vi "Middfield_171213.vi"(8 "StartingAngle":i16, 9 "DiameterOfTheMidfield":u16, 10 "Midfield":enum16{"4", "3", "2", "1", "0"}(ring), 11 "InputBackground":picture) -> (2 "Colors":u32[](array[numeric]), 3 "OutputBackground":picture)   [LabVIEW 2016]
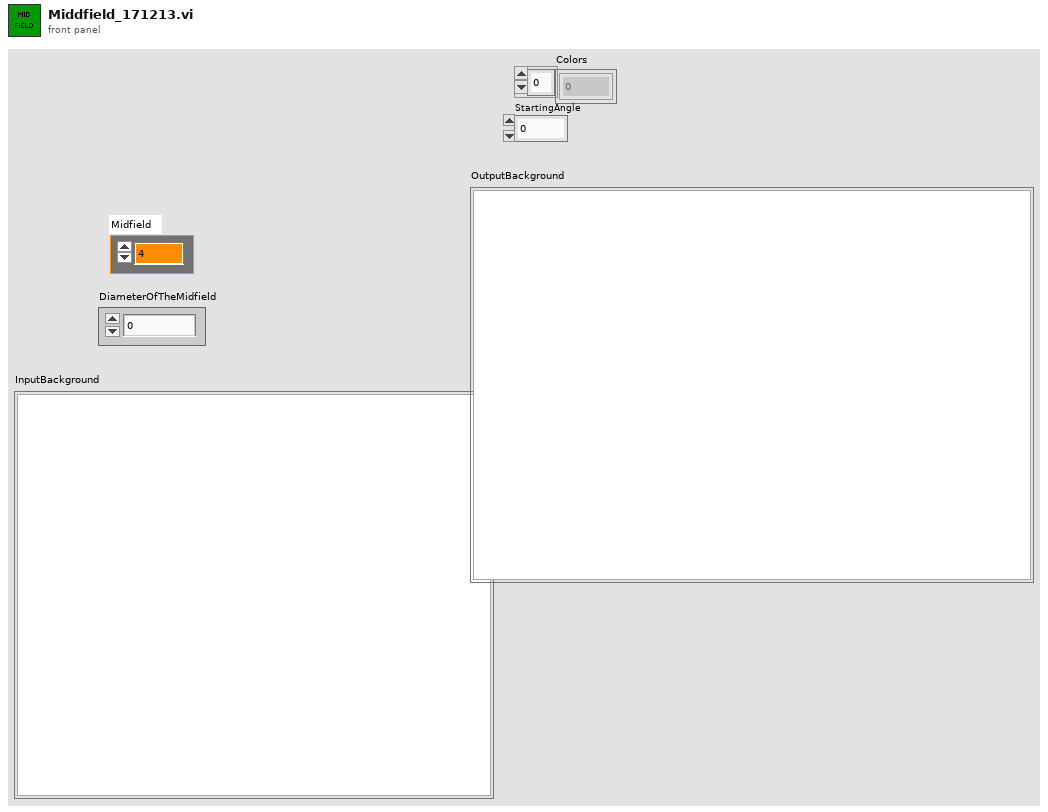
[diagram p1: front panel]
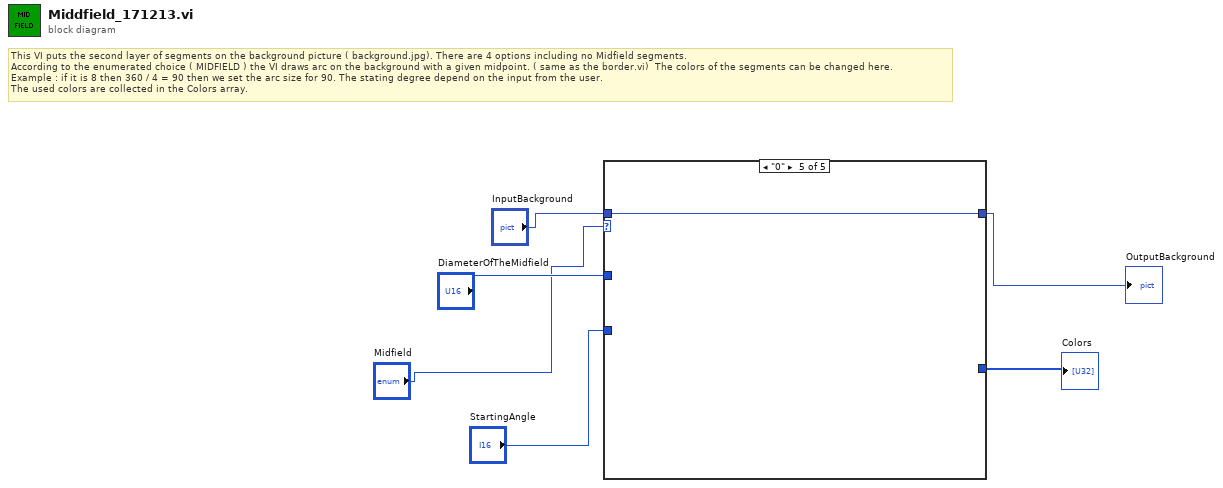
[diagram p0: block diagram]
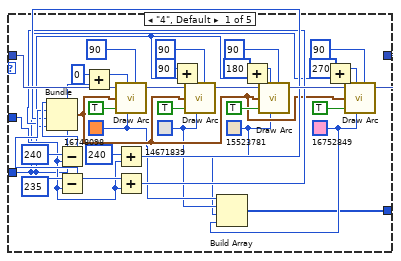
[diagram p2: hidden frame]
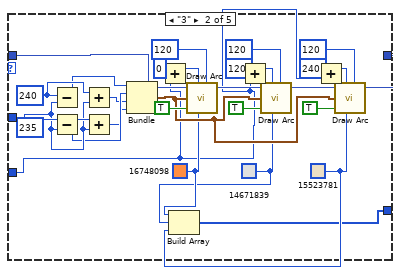
[diagram p3: hidden frame]
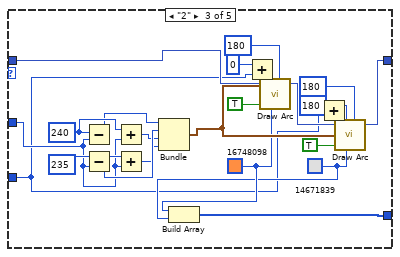
[diagram p4: hidden frame]
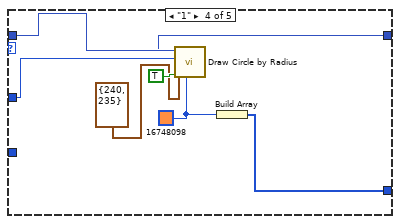
[diagram p5: hidden frame]
diagram:
  # "This VI puts the second layer of segments on the background picture ( background.jpg). There are 4 options including no Midfield segments.\nAccording to the enumerated choice ( MIDFIELD ) the VI draws arc on the background with a given midpoint. ( same as the border.vi)  The colors of the segments can be changed here. \nExample : if it is 8 then 360 / 4 = 90 then we set the arc size for 90. The stating degree depend on the input from the user. \nThe used colors are collected in the Colors array."
  n1 = case shown="\"0\"" "Midfield" {
    tunnel: [w26 w59 w86 w98 w102] -> w6
    tunnel: "InputBackground" -> [w31 w64 w91 w99 w102]
    tunnel: "DiameterOfTheMidfield" -> [w20 w56 w78 w97 _]
    tunnel: "StartingAngle" -> [w8 w44 w73 _ _]
    tunnel: [w7 w43 w72 w95 _] -> w1
    frame "4", Default {
      w21 = i16 235 ("vertical")
      w13 = u32 16752849 ("color(black)")
      w14 = u32 15523781 ("color(black)")
      w15 = u32 14671839 ("color(black)")
      w16 = u32 16748098 ("color(black)")
      n2 = Subtract(x=i16 240 ("horizontal"), y=w20) -> (x-y=w24:u16)
      n3 = Subtract(x=w21, y=w20) -> (x-y=w23:u16)
      n4 = Add(x=i16 0 ("start angle[degrees]"), y=w8) -> (x+y=w12:i16)
      n5 = Add(x=i16 240 ("horizontal"), y=w20) -> (x+y=w19:u16)
      n6 = Add(x=w21, y=w20) -> (x+y=w18:u16)
      n7 = Bundle(w24, w23, w19, w18) -> (w17:cluster{u16, u16, u16, u16})  [unwired: 1 in]
      n8 = call <vilib>:"Draw Arc.vi"("picture"=w31, "start angle[degrees]"=w12, "rect"=w17, "fill?(F)"=TRUE, "color(black)"=w16, "arc size[degrees]"=i16 90) -> ("new picture"=w36:picture)  [unwired: 3 in]
      n9 = Add(x=i16 90 ("start angle[degrees]"), y=w8) -> (x+y=w11:i16)
      n10 = call <vilib>:"Draw Arc.vi"("picture"=w36, "start angle[degrees]"=w11, "rect"=w17, "fill?(F)"=TRUE, "color(black)"=w15, "arc size[degrees]"=i16 90) -> ("new picture"=w32:picture)  [unwired: 3 in]
      n11 = Build Array(w16, w15, w14, w13) -> (w7:u32[])
      n12 = Add(x=i16 180 ("start angle[degrees]"), y=w8) -> (x+y=w10:i16)
      n13 = call <vilib>:"Draw Arc.vi"("picture"=w32, "start angle[degrees]"=w10, "rect"=w17, "fill?(F)"=TRUE, "color(black)"=w14, "arc size[degrees]"=i16 90) -> ("new picture"=w27:picture)  [unwired: 3 in]
      n14 = Add(x=i16 270 ("start angle[degrees]"), y=w8) -> (x+y=w9:i16)
      n15 = call <vilib>:"Draw Arc.vi"("picture"=w27, "start angle[degrees]"=w9, "rect"=w17, "fill?(F)"=TRUE, "color(black)"=w13, "arc size[degrees]"=i16 90) -> ("new picture"=w26:picture)  [unwired: 3 in]
    }
    frame "3" {
      w57 = i16 235 ("vertical")
      w58 = i16 240 ("horizontal")
      w48 = u32 15523781 ("color(black)")
      w49 = u32 14671839 ("color(black)")
      w50 = u32 16748098 ("color(black)")
      n16 = Subtract(x=w58, y=w56) -> (x-y=w55:u16)
      n17 = Subtract(x=w57, y=w56) -> (x-y=w54:u16)
      n18 = Add(x=w58, y=w56) -> (x+y=w52:u16)
      n19 = Add(x=w57, y=w56) -> (x+y=w53:u16)
      n20 = Bundle(w55, w54, w52, w53) -> (w51:cluster{u16, u16, u16, u16})  [unwired: 1 in]
      n21 = Add(x=i16 0 ("start angle[degrees]"), y=w44) -> (x+y=w47:i16)
      n22 = Build Array(w50, w49, w48) -> (w43:u32[])
      n23 = call <vilib>:"Draw Arc.vi"("picture"=w64, "start angle[degrees]"=w47, "rect"=w51, "fill?(F)"=TRUE, "color(black)"=w50, "arc size[degrees]"=i16 120) -> ("new picture"=w65:picture)  [unwired: 3 in]
      n24 = Add(x=i16 120 ("start angle[degrees]"), y=w44) -> (x+y=w46:i16)
      n25 = call <vilib>:"Draw Arc.vi"("picture"=w65, "start angle[degrees]"=w46, "rect"=w51, "fill?(F)"=TRUE, "color(black)"=w49, "arc size[degrees]"=i16 120) -> ("new picture"=w60:picture)  [unwired: 3 in]
      n26 = Add(x=i16 240 ("start angle[degrees]"), y=w44) -> (x+y=w45:i16)
      n27 = call <vilib>:"Draw Arc.vi"("picture"=w60, "start angle[degrees]"=w45, "rect"=w51, "fill?(F)"=TRUE, "color(black)"=w48, "arc size[degrees]"=i16 120) -> ("new picture"=w59:picture)  [unwired: 3 in]
    }
    frame "2" {
      w84 = i16 235 ("vertical")
      w85 = i16 240 ("horizontal")
      w76 = u32 14671839 ("color(black)")
      w77 = u32 16748098 ("color(black)")
      n28 = Subtract(x=w85, y=w78) -> (x-y=w83:u16)
      n29 = Subtract(x=w84, y=w78) -> (x-y=w82:u16)
      n30 = Add(x=w85, y=w78) -> (x+y=w80:u16)
      n31 = Add(x=w84, y=w78) -> (x+y=w81:u16)
      n32 = Bundle(w83, w82, w80, w81) -> (w79:cluster{u16, u16, u16, u16})  [unwired: 1 in]
      n33 = Build Array(w77, w76) -> (w72:u32[])
      n34 = Add(x=i16 0 ("start angle[degrees]"), y=w73) -> (x+y=w75:i16)
      n35 = call <vilib>:"Draw Arc.vi"("picture"=w91, "start angle[degrees]"=w75, "rect"=w79, "fill?(F)"=TRUE, "color(black)"=w77, "arc size[degrees]"=i16 180) -> ("new picture"=w87:picture)  [unwired: 3 in]
      n36 = Add(x=i16 180 ("start angle[degrees]"), y=w73) -> (x+y=w74:i16)
      n37 = call <vilib>:"Draw Arc.vi"("picture"=w87, "start angle[degrees]"=w74, "rect"=w79, "fill?(F)"=TRUE, "color(black)"=w76, "arc size[degrees]"=i16 180) -> ("new picture"=w86:picture)  [unwired: 3 in]
    }
    frame "1" {
      w96 = u32 16748098 ("color(black)")
      n38 = call <vilib>:"Draw Circle by Radius.vi"("color(black)"=w96, "fill?(F)"=TRUE, "pixel center"=cluster{"horizontal":i16, "vertical":i16} {"horizontal"=240, "vertical"=235}, "radius"=w97, "picture"=w99) -> ("new picture"=w98:picture)  [unwired: 6 in]
      n39 = Build Array(w96) -> (w95:u32[])
    }
    frame "0" {
    }
  }
  "OutputBackground" <- w6
  "Colors" <- w1
